vi "Begin.vi"(8 "error in":errorcluster) -> (0 "error out":errorcluster)   [LabVIEW 2016]
doc: "Called before other user functions, this VI is expected to open initial I/O refnums, load in file data, and do all program initialization. Notice that the <B>error out</B> terminal is simply used for data flow. Wiring it to other structures or subVIs ensures that this VI runs first."
uses:
  <vilib>/Rock Robotics/WPI/DriverStation/WPI_DriverStationRobotMode2.ctl
  <vilib>/Rock Robotics/WPI/Joystick/WPI_JoystickDeviceEnum.ctl
  <vilib>/Rock Robotics/SystemInterfaces/DIO/FPGA_DIORelayChannel.ctl
  Robot Global Data.vi
  <vilib>/Rock Robotics/Network Tables/NT Write String Array.vi
  <vilib>/Rock Robotics/WPI/RobotDrive/WPI_RobotDriveOpen4MotorWithExistingMotors.vi
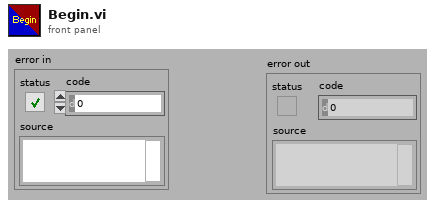
[diagram p1: front panel]
types:
  T1 = typedef "FPGA_DIORelayChannel.ctl" = enum8{"Relay 0", "Relay 1", "Relay 2", "Relay 3", "Invalid"}
  T2 = typedef "WPI_JoystickDeviceEnum.ctl" = enum16{"USB 0", "USB 1", "USB 2", "USB 3", "USB 4", "USB 5"}
  T3 = typedef "WPI_DriverStationRobotMode2.ctl" = enum16{"Autonomous Disabled", "Autonomous Enabled", "Teleop Disabled", "Teleop Enabled", "Disconnected", "Finish", "Test Disabled", "Test Enabled", "Emergency Stopped"}
  T4 = typedef "WPI_MotorControlDeviceRef.ctl" = cluster{"DeviceStatus":errorcluster, "Type":T5, "PWM":cluster{"PWM Channel":T6, "DeadBand":T7}, "CAN":cluster{"Device Number":u8, "SetOutput VI Ref":variant, "GetOutput VI Ref":variant, "Enable VI Ref":variant, "Disable VI Ref":variant, "Data":variant}, "Invert":bool}
  T5 = typedef "WPI_MotorControlType.ctl" = enum16{"PWM", "CAN"}
  T6 = typedef "FPGA_DIOPWMChannel.ctl" = enum8{"PWM 0", "PWM 1", "PWM 2", "PWM 3", "PWM 4", "PWM 5", "PWM 6", "PWM 7", "PWM 8", "PWM 9", "PWM MXP 0", "PWM MXP 1", "PWM MXP 2", "PWM MXP 3", "PWM MXP 4", "PWM MXP 5", "PWM MXP 6", "PWM MXP 7", "PWM MXP 8", "PWM MXP 9", "Invalid"}
  T7 = typedef "WPI_PWMDeadband.ctl" = cluster{"Name":string, "maxPositivePwm":i32, "minPositivePwm":i32, "centerPwm":i32, "maxNegativePwm":i32, "minNegativePwm":i32, "angularRange":u16}
  T8 = typedef "WPI_JoystickDevRef.ctl" = cluster{"Device":T2}
  T9 = typedef "WPI_RobotDriveDevRef.ctl" = cluster{"DevStatus":errorcluster, "Motors[]":T4[], "Square Inputs":bool, "Max Output":dbl}
  T10 = typedef "WPI_RelayDevRef.ctl" = cluster{"DevStatus":errorcluster, "Relay Channel":T1, "Relay Direction":T11}
  T11 = typedef "WPI_RelayDirection.ctl" = enum16{"Both directions", "Forward only", "Reverse only"}
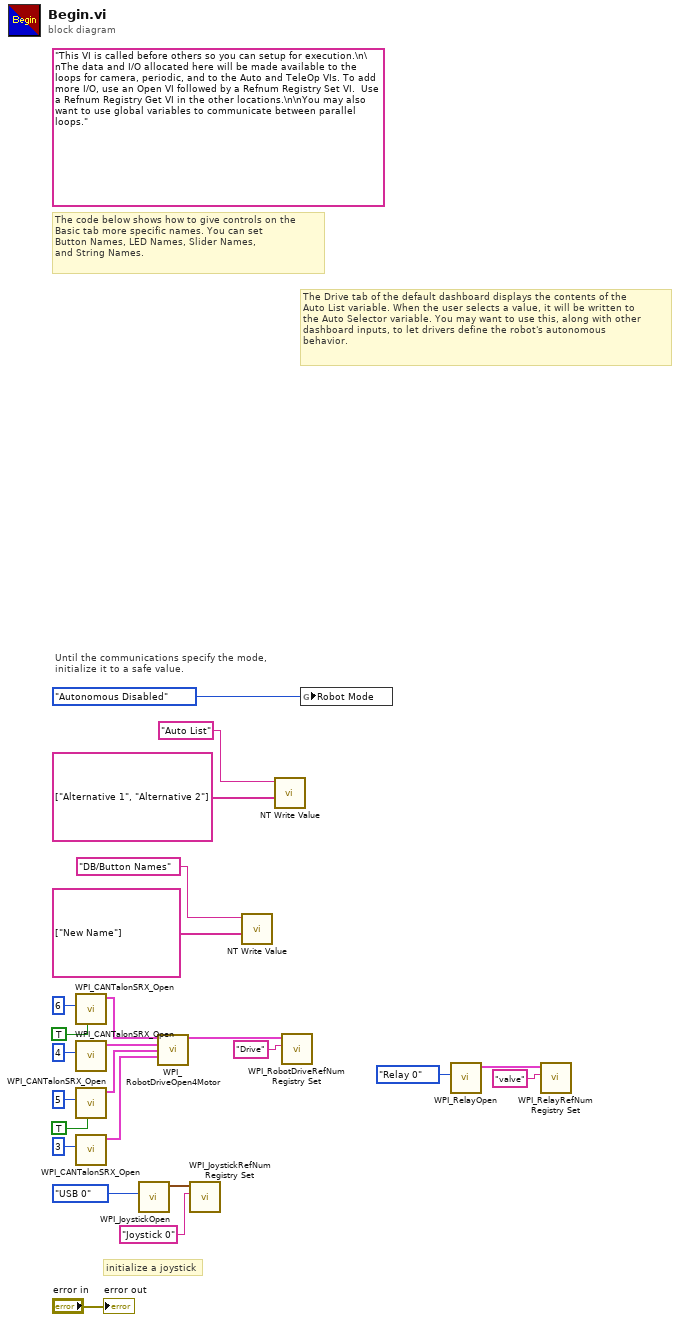
[diagram p0: block diagram]
diagram:
  (unwired) "This VI is called before others so you can setup for execution.\n\nThe data and I/O allocated here will be made available to the loops for camera, periodic, and to the Auto and TeleOp VIs. To add more I/O, use an Open VI followed by a Refnum Registry Set VI.  Use a Refnum Registry Get VI in the other locations.\n\nYou may also want to use global variables to communicate between parallel loops."
  # "The Drive tab of the default dashboard displays the contents of the\nAuto List variable. When the user selects a value, it will be written to\nthe Auto Selector variable. You may want to use this, along with other\ndashboard inputs, to let drivers define the robot's autonomous\nbehavior."
  # "The code below shows how to give controls on the\nBasic tab more specific names. You can set\nButton Names, LED Names, Slider Names,\nand String Names."
  # "initialize a joystick"
  # "Until the communications specify the mode,\ninitialize it to a safe value."
  n1 = call <vilib>:"WPI_CANTalonSRX_Open.vi"("Invert"=TRUE, "Device Number"=u8 6) -> ("CAN Talon SRX Ref"=w15:T4)  [unwired: 8 in, 1 out]
  n2 = call <vilib>:"WPI_CANTalonSRX_Open.vi"("Device Number"=u8 4) -> ("CAN Talon SRX Ref"=w14:T4)  [unwired: 9 in, 1 out]
  n3 = call <vilib>:"WPI_CANTalonSRX_Open.vi"("Invert"=TRUE, "Device Number"=u8 5) -> ("CAN Talon SRX Ref"=w13:T4)  [unwired: 8 in, 1 out]
  n4 = call <vilib>:"WPI_CANTalonSRX_Open.vi"("Device Number"=u8 3) -> ("CAN Talon SRX Ref"=w12:T4)  [unwired: 9 in, 1 out]
  n5 = call <vilib>:"WPI_JoystickOpen.vi"("JoystickDevice"=WPI_JoystickDeviceEnum."USB 0") -> ("JoystickDevRef"=w22:T8)  [unwired: 10 in]
  n6 = call-poly <vilib>:"WPI_RobotDriveOpen4Motor.vi"("Rear Left Motor Dev Ref"=w15, "Rear Right Motor Dev Ref"=w14, "Front Left Motor Dev Ref"=w13, "Front Right Motor Dev Ref"=w12) -> ("RobotDriveDevRef"=w7:T9)  [unwired: 10 in, 1 out]
  n7 = call <vilib>:"WPI_JoystickRefNum Registry Set.vi"("refnum name"="Joystick 0", "JoystickDevRef"=w22) -> ()  [unwired: 8 in, 2 out]
  n8 = call-poly <vilib>:"NT Write Value.vi"("String Array"=string[] ["New Name"], "Name"="DB/Button Names") -> ()  [unwired: 9 in, 1 out]
  n9 = call-poly <vilib>:"NT Write Value.vi"("String Array"=string[] ["Alternative 1", "Alternative 2"], "Name"="Auto List") -> ()  [unwired: 9 in, 1 out]
  n10 = call <vilib>:"WPI_RobotDriveRefNum Registry Set.vi"("refnum name"="Drive", "RobotDriveDevRef"=w7) -> ()  [unwired: 8 in, 2 out]
  n11 = global write "Robot Global Data.vi" "Robot Mode"(WPI_DriverStationRobotMode2."Autonomous Disabled" ("Robot Mode")) -> ()
  n12 = call <vilib>:"WPI_RelayOpen.vi"("Relay Channel"=FPGA_DIORelayChannel."Relay 0") -> ("RelayDevRef"=w3:T10)  [unwired: 9 in, 1 out]
  n13 = call <vilib>:"WPI_RelayRefNum Registry Set.vi"("refnum name"="valve", "RelayDevRef"=w3) -> ()  [unwired: 8 in, 2 out]
  "error out" <- "error in"
